vi "FreshScroll.vi"(8 "error in (no error)":errorcluster, 9 "Index":u32, 10 "Scroll":refnum<vi>, 11 "Scroller.lvclass":refnum<class "Scroller.lvclass">) -> (0 "error out":errorcluster, 3 "Scroller.lvclass out":refnum<class "Scroller.lvclass">)   [LabVIEW 2015, in "ActorManagement.lvlib" / "Scroller.lvclass"]
uses:
  Scroller.lvclass
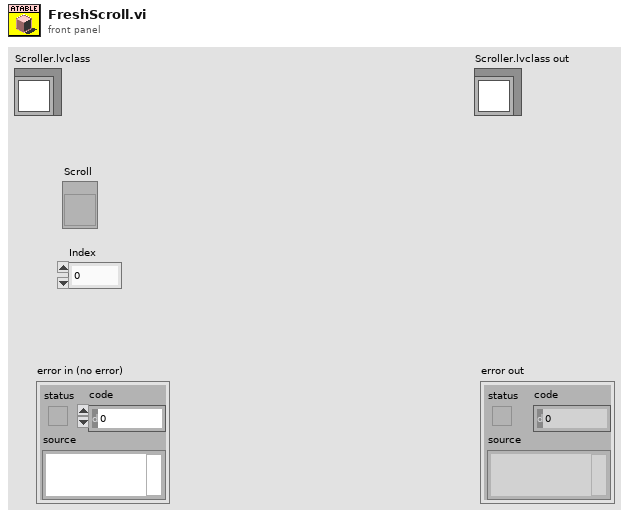
[diagram p1: front panel]
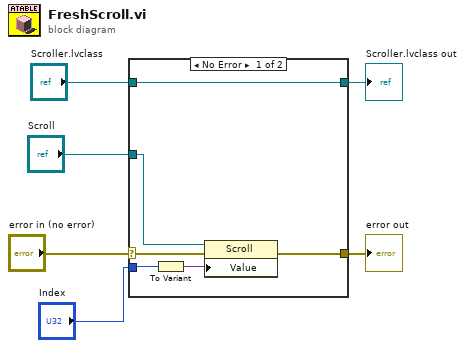
[diagram p0: block diagram]
diagram:
  n1 = case shown="No Error" "error in (no error)" {
    selector: "error in (no error)" -> [w12 w14]
    tunnel: [w11 w14] -> w5
    tunnel: "Scroller.lvclass" -> [w9 w13]
    tunnel: "Scroll" -> [w10 _]
    tunnel: "Index" -> [w8 _]
    tunnel: [w9 w13] -> w2
    frame No Error {
      n2 = To Variant(anything=w8) -> (Variant=w7:variant)
      n3 = property class="Scroll"(reference=w10, error in=w12, "Value"=w7) -> (error out=w11:errorcluster)  [unwired: 1 out]
    }
    frame Error {
    }
  }
  "error out" <- w5
  "Scroller.lvclass out" <- w2
